vi "Update Value Control.vi"(0 "Session In":T2, 1 "Force update?":bool, 5 "Tree Control In":refnum<vi>, 7 "Tab Control Ref In":T1, 11 "error in (no error)":errorcluster) -> (4 "Session Out":T2, 6 "Tree Control Out":refnum<vi>, 8 "Units":string, 10 "Tooltip":string, 15 "error out":errorcluster)   [LabVIEW 2009, in "IMAQdx Cam.lvclass"]
doc: "The Update Value Control subVI determines the type of the attribute selected, displays the corresponding tab in the tab control, sets the current value of the control, sets the minimum and maximum of the control (for numerics), and disables the control if the attribute is not writables."
uses:
  IMAQdx Cam.lvclass
  <vilib>/userDefined/High Color/IMAQdx.ctl
  <vilib>/vision/driver/IMAQdx.llb/IMAQdx Attribute Type.ctl
  <vilib>/vision/driver/NI_Vision_Acquisition_Software.lvlib
  C:/Program Files/National Instruments/LabVIEW 2009/resource/objmgr/imaqdx.rc
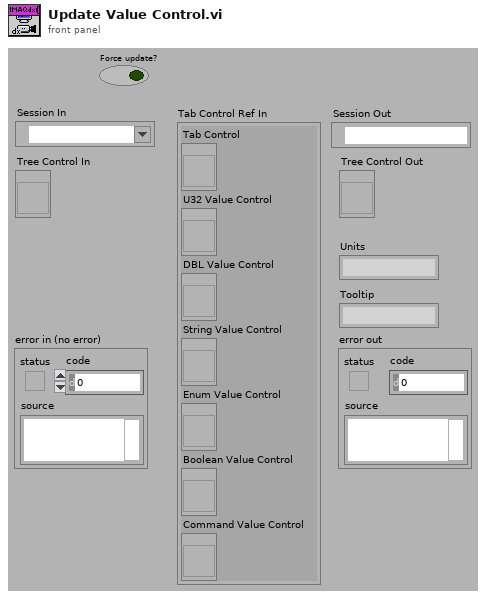
[diagram p1: front panel]
types:
  T1 = cluster{"Tab Control":refnum<vi>, "U32 Value Control":refnum<vi>, "DBL Value Control":refnum<vi>, "String Value Control":refnum<vi>, "Enum Value Control":refnum<vi>, "Boolean Value Control":refnum<vi>, "Command Value Control":refnum<vi>}
  T2 = typedef "IMAQdx.ctl" = refnum<k21>
  T3 = typedef "NI_Vision_Acquisition_Software.lvlib/IMAQdx Attribute Type.ctl" = enum32{"U32", "I64", "DBL", "String", "Enum", "Bool", "Command"}
  T4 = enum32{"U32", "DBL", "String", "Enum", "Bool", "Command"}
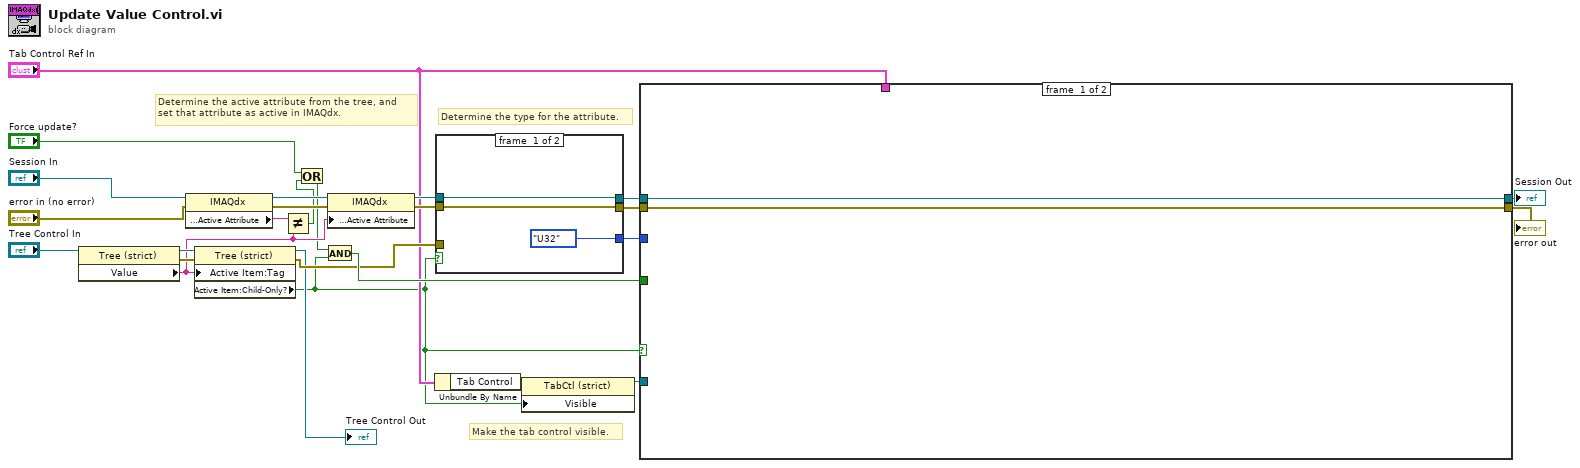
[diagram p0: block diagram]
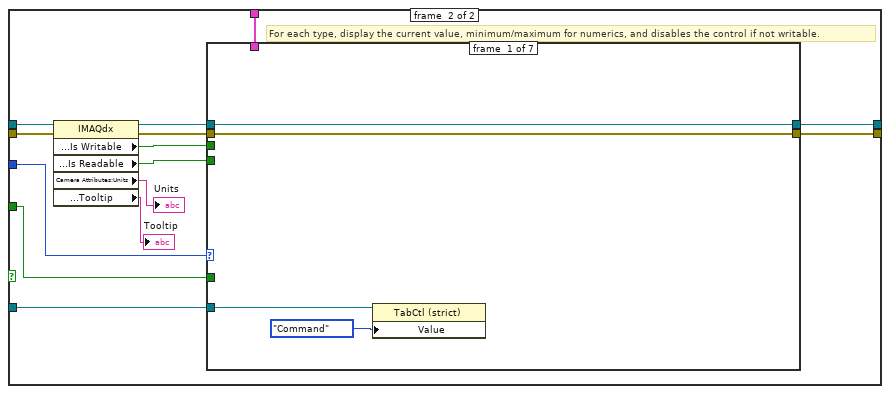
[diagram p2: hidden frame]
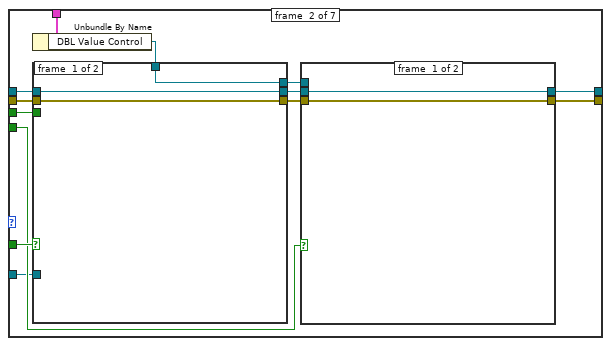
[diagram p3: hidden frame]
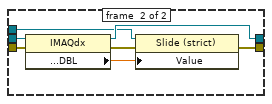
[diagram p4: hidden frame]
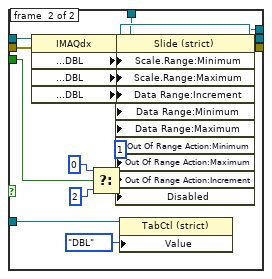
[diagram p5: hidden frame]
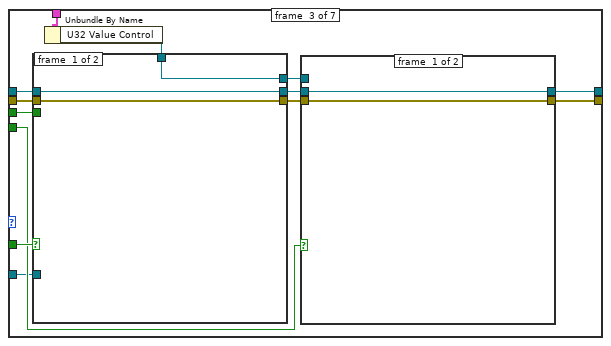
[diagram p6: hidden frame]
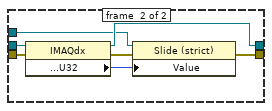
[diagram p7: hidden frame]
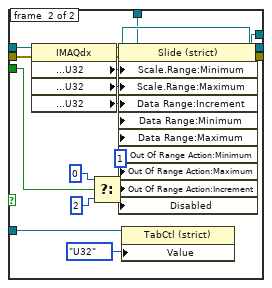
[diagram p8: hidden frame]
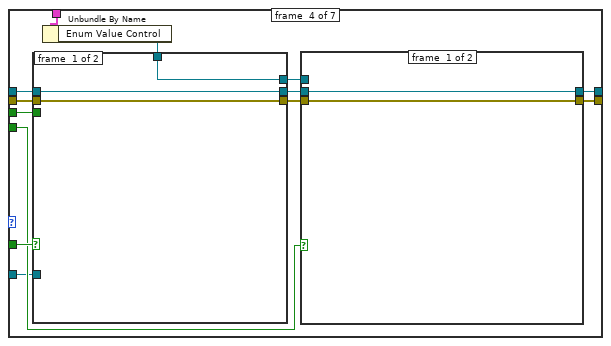
[diagram p9: hidden frame]
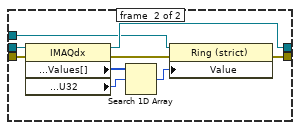
[diagram p10: hidden frame]
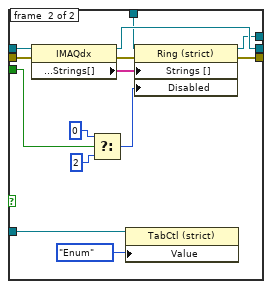
[diagram p11: hidden frame]
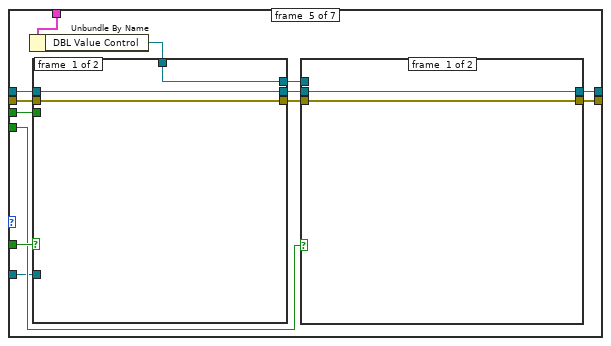
[diagram p12: hidden frame]
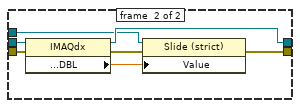
[diagram p13: hidden frame]
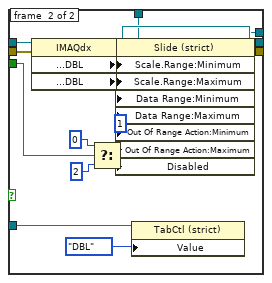
[diagram p14: hidden frame]
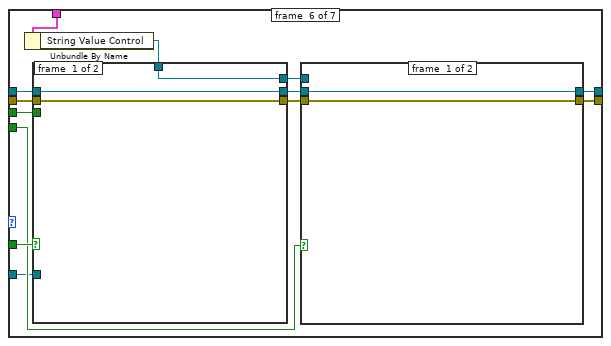
[diagram p15: hidden frame]
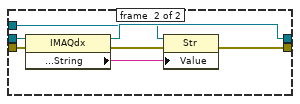
[diagram p16: hidden frame]
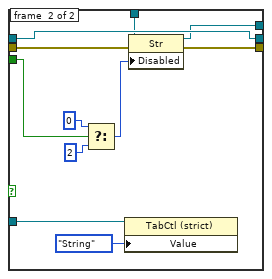
[diagram p17: hidden frame]
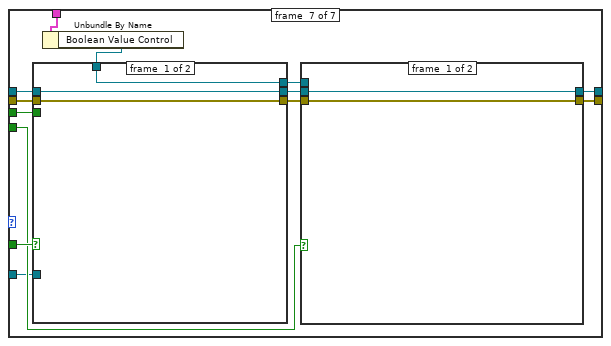
[diagram p18: hidden frame]
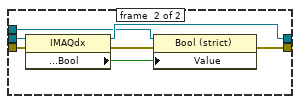
[diagram p19: hidden frame]
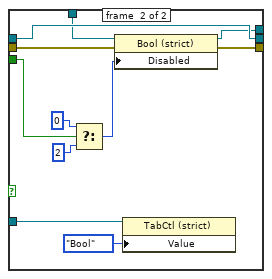
[diagram p20: hidden frame]
diagram:
  # "Make the tab control visible."
  # "Determine the type for the attribute."
  # "Determine the active attribute from the tree, and \nset that attribute as active in IMAQdx."
  n1 = property class="Tree (strict)"(reference="Tree Control In") -> (reference out=w11:refnum<vi>, error out=w10:errorcluster, "Value"=w9:string)  [unwired: 1 in]
  n2 = property class="IMAQdx"(reference="Session In", error in="error in (no error)") -> (reference out=w25:T2, error out=w24:errorcluster, "Camera Attributes:Active Attribute"=w26:string)
  n3 = property class="Tree (strict)"(reference=w11, error in=w10, "Active Item:Tag"=w9) -> (reference out=→"Tree Control Out":refnum<vi>, error out=w17:errorcluster, "Active Item:Child-Only?"=w5:bool)
  n4 = Not Equal?(x=w26, y=w9) -> (x != y?=w3:bool)
  n5 = Or(x="Force update?", y=w3) -> (x .or. y?=w1:bool)
  n6 = And(x=w1, y=w5) -> (x .and. y?=w18:bool)
  n7 = property class="IMAQdx"(reference=w25, error in=w24, "Camera Attributes:Active Attribute"=w9) -> (reference out=w23:T2, error out=w22:errorcluster)
  n8 = Unbundle By Name("Tab Control Ref In") -> ("Tab Control"=w7:refnum<vi>)
  n9 = case shown="True" w5 {
    tunnel: w23 -> [w29 w36]
    tunnel: [w29 w33] -> w20
    tunnel: [IMAQdx_Attribute_Type."U32" ("Attribute Type") w32] -> w19
    tunnel: w22 -> [w27 w31]
    tunnel: [w27 w30] -> w21
    tunnel: w17 -> [_ _]
    frame #0 {
    }
    frame #1 {
      n10 = property class="IMAQdx"(reference=w36, error in=w31) -> (reference out=w33:T2, error out=w30:errorcluster, "Camera Attributes:Type"=w35:u32)
      n11 = Type Cast(type=IMAQdx_Attribute_Type."U32" ("Attribute Type"), x=w35) -> (*(type *) &x=w32:T3)
    }
  }
  n12 = property class="TabCtl (strict)"(reference=w7, "Visible"=w5) -> (reference out=w4:refnum<vi>)  [unwired: 1 in, 1 out]
  n13 = case shown="True" w5 {
    tunnel: w21 -> [w38 w51]
    tunnel: [w38 w43] -> w12
    tunnel: w20 -> [w37 w52]
    tunnel: w19 -> [_ w49]
    tunnel: w18 -> [_ w44]
    tunnel: [w37 w42] -> w13
    tunnel: "Tab Control Ref In" -> [_ w41]
    tunnel: w4 -> [_ w40]
    frame #0 {
    }
    frame #1 {
      # "For each type, display the current value, minimum/maximum for numerics, and disables the control if not writable."
      n14 = property class="IMAQdx"(reference=w52, error in=w51) -> (reference out=w46:T2, error out=w45:errorcluster, "Camera Attributes:Is Writable"=w48:bool, "Camera Attributes:Is Readable"=w47:bool, "Camera Attributes:Units"=→"Units":string, "Camera Attributes:Tooltip"=→"Tooltip":string)
      n15 = case shown="\"DBL\"" w49 {
        tunnel: w48 -> [_ w66 w108 w150 w191 w232 w268]
        tunnel: w47 -> [_ w65 w107 w149 w190 w231 w267]
        tunnel: w46 -> [w55 w69 w111 w153 w194 w235 w271]
        tunnel: w45 -> [w56 w68 w110 w152 w193 w234 w270]
        tunnel: w44 -> [_ w67 w109 w151 w192 w233 w269]
        tunnel: [w56 w62 w104 w146 w187 w228 w264] -> w43
        tunnel: [w55 w61 w103 w145 w186 w227 w263] -> w42
        tunnel: w41 -> [_ w59 w100 w142 w185 w225 w261]
        tunnel: w40 -> [w54 w60 w101 w143 w183 w226 w262]
        frame #0 {
          n16 = property class="TabCtl (strict)"(reference=w54, "Value"=T4."Command" ("Tab Control")) -> ()  [unwired: 1 in, 2 out]
        }
        frame #1 {
          n17 = Unbundle By Name(w59) -> ("DBL Value Control"=w58:refnum<vi>)
          n18 = case shown="True" w67 {
            tunnel: w69 -> [w81 w98]
            tunnel: w68 -> [w80 w97]
            tunnel: [w81 w91] -> w64
            tunnel: [w80 w87] -> w63
            tunnel: w66 -> [_ w96]
            tunnel: w60 -> [_ w93]
            tunnel: w58 -> [w79 w89]
            tunnel: [w79 w88] -> w57
            frame #0 {
            }
            frame #1 {
              w83 = u8 1 ("Out Of Range Action:Maximum")
              n19 = property class="IMAQdx"(reference=w98, error in=w97) -> (reference out=w91:T2, error out=w90:errorcluster, "Camera Attributes:Minimum:DBL"=w85:dbl, "Camera Attributes:Maximum:DBL"=w84:dbl, "Camera Attributes:Increment:DBL"=w82:dbl)
              n20 = Select(t=0, s=w96, f=2) -> (s? t:f=w86:i32)
              n21 = property class="Slide (strict)"(reference=w89, error in=w90, "Scale.Range:Minimum"=w85, "Scale.Range:Maximum"=w84, "Data Range:Increment"=w82, "Data Range:Minimum"=w85, "Data Range:Maximum"=w84, "Out Of Range Action:Minimum"=w83, "Out Of Range Action:Maximum"=w83, "Out Of Range Action:Increment"=w83, "Disabled"=w86) -> (reference out=w88:refnum<vi>, error out=w87:errorcluster)
              n22 = property class="TabCtl (strict)"(reference=w93, "Value"=T4."DBL" ("Tab Control")) -> ()  [unwired: 1 in, 2 out]
            }
          }
          n23 = case shown="True" w65 {
            tunnel: w64 -> [w71 w78]
            tunnel: w63 -> [w70 w77]
            tunnel: [w71 w75] -> w61
            tunnel: [w70 w76] -> w62
            tunnel: w57 -> [_ w73]
            frame #0 {
            }
            frame #1 {
              n24 = property class="IMAQdx"(reference=w78, error in=w77) -> (reference out=w75:T2, error out=w74:errorcluster, "Camera Attributes:Value:DBL"=w72:dbl)
              n25 = property class="Slide (strict)"(reference=w73, error in=w74, "Value"=w72) -> (error out=w76:errorcluster)  [unwired: 1 out]
            }
          }
        }
        frame #2 {
          n26 = Unbundle By Name(w100) -> ("U32 Value Control"=w99:refnum<vi>)
          n27 = case shown="True" w109 {
            tunnel: w111 -> [w123 w140]
            tunnel: w110 -> [w122 w139]
            tunnel: [w123 w134] -> w106
            tunnel: [w122 w132] -> w105
            tunnel: w108 -> [_ w138]
            tunnel: [w121 w131] -> w102
            tunnel: w101 -> [_ w130]
            tunnel: w99 -> [w121 w128]
            frame #0 {
            }
            frame #1 {
              w127 = u8 1 ("Out Of Range Action:Maximum")
              n28 = property class="IMAQdx"(reference=w140, error in=w139) -> (reference out=w134:T2, error out=w135:errorcluster, "Camera Attributes:Minimum:U32"=w125:u32, "Camera Attributes:Maximum:U32"=w124:u32, "Camera Attributes:Increment:U32"=w126:u32)
              n29 = Select(t=0, s=w138, f=2) -> (s? t:f=w133:i32)
              n30 = property class="Slide (strict)"(reference=w128, error in=w135, "Scale.Range:Minimum"=w125, "Scale.Range:Maximum"=w124, "Data Range:Increment"=w126, "Data Range:Minimum"=w125, "Data Range:Maximum"=w124, "Out Of Range Action:Minimum"=w127, "Out Of Range Action:Maximum"=w127, "Out Of Range Action:Increment"=w127, "Disabled"=w133) -> (reference out=w131:refnum<vi>, error out=w132:errorcluster)
              n31 = property class="TabCtl (strict)"(reference=w130, "Value"=T4."U32" ("Tab Control")) -> ()  [unwired: 1 in, 2 out]
            }
          }
          n32 = case shown="True" w107 {
            tunnel: w106 -> [w113 w120]
            tunnel: w105 -> [w112 w119]
            tunnel: [w113 w118] -> w103
            tunnel: [w112 w114] -> w104
            tunnel: w102 -> [_ w115]
            frame #0 {
            }
            frame #1 {
              n33 = property class="IMAQdx"(reference=w120, error in=w119) -> (reference out=w118:T2, error out=w117:errorcluster, "Camera Attributes:Value:U32"=w116:u32)
              n34 = property class="Slide (strict)"(reference=w115, error in=w117, "Value"=w116) -> (error out=w114:errorcluster)  [unwired: 1 out]
            }
          }
        }
        frame #3 {
          n35 = Unbundle By Name(w142) -> ("Enum Value Control"=w141:refnum<vi>)
          n36 = case shown="True" w151 {
            tunnel: w153 -> [w167 w181]
            tunnel: w152 -> [w166 w180]
            tunnel: [w167 w176] -> w148
            tunnel: [w166 w174] -> w147
            tunnel: w150 -> [_ w179]
            tunnel: [w165 w173] -> w144
            tunnel: w143 -> [_ w170]
            tunnel: w141 -> [w165 w168]
            frame #0 {
            }
            frame #1 {
              n37 = property class="IMAQdx"(reference=w181, error in=w180) -> (reference out=w176:T2, error out=w175:errorcluster, "Camera Attributes:Enum:Strings[]"=w171:string[])
              n38 = Select(t=0, s=w179, f=2) -> (s? t:f=w172:i32)
              n39 = property class="TabCtl (strict)"(reference=w170, "Value"=T4."Enum" ("Tab Control")) -> ()  [unwired: 1 in, 2 out]
              n40 = property class="Ring (strict)"(reference=w168, error in=w175, "Strings []"=w171, "Disabled"=w172) -> (reference out=w173:refnum<vi>, error out=w174:errorcluster)
            }
          }
          n41 = case shown="True" w149 {
            tunnel: w148 -> [w155 w164]
            tunnel: w147 -> [w154 w163]
            tunnel: [w155 w158] -> w145
            tunnel: [w154 w160] -> w146
            tunnel: w144 -> [_ w157]
            frame #0 {
            }
            frame #1 {
              n42 = property class="IMAQdx"(reference=w164, error in=w163) -> (reference out=w158:T2, error out=w156:errorcluster, "Camera Attributes:Enum:Values[]"=w162:u32[], "Camera Attributes:Value:U32"=w161:u32)
              n43 = Search 1D Array(1D array=w162, element=w161) -> (index of element=w159:i32)  [unwired: 1 out]
              n44 = property class="Ring (strict)"(reference=w157, error in=w156, "Value"=w159) -> (error out=w160:errorcluster)  [unwired: 1 out]
            }
          }
        }
        frame #4 {
          n45 = Unbundle By Name(w185) -> ("DBL Value Control"=w184:refnum<vi>)
          n46 = case shown="True" w192 {
            tunnel: w194 -> [w206 w222]
            tunnel: w193 -> [w205 w221]
            tunnel: [w206 w217] -> w189
            tunnel: [w205 w212] -> w188
            tunnel: w191 -> [_ w220]
            tunnel: w184 -> [w204 w215]
            tunnel: [w204 w214] -> w182
            tunnel: w183 -> [_ w211]
            frame #0 {
            }
            frame #1 {
              w207 = u8 1 ("Out Of Range Action:Minimum")
              n47 = property class="IMAQdx"(reference=w222, error in=w221) -> (reference out=w217:T2, error out=w216:errorcluster, "Camera Attributes:Minimum:DBL"=w209:dbl, "Camera Attributes:Maximum:DBL"=w208:dbl)
              n48 = Select(t=0, s=w220, f=2) -> (s? t:f=w213:i32)
              n49 = property class="Slide (strict)"(reference=w215, error in=w216, "Scale.Range:Minimum"=w209, "Scale.Range:Maximum"=w208, "Data Range:Minimum"=w209, "Data Range:Maximum"=w208, "Out Of Range Action:Minimum"=w207, "Out Of Range Action:Maximum"=w207, "Disabled"=w213) -> (reference out=w214:refnum<vi>, error out=w212:errorcluster)
              n50 = property class="TabCtl (strict)"(reference=w211, "Value"=T4."DBL" ("Tab Control")) -> ()  [unwired: 1 in, 2 out]
            }
          }
          n51 = case shown="True" w190 {
            tunnel: w189 -> [w196 w203]
            tunnel: w188 -> [w195 w202]
            tunnel: [w196 w201] -> w186
            tunnel: [w195 w199] -> w187
            tunnel: w182 -> [_ w198]
            frame #0 {
            }
            frame #1 {
              n52 = property class="IMAQdx"(reference=w203, error in=w202) -> (reference out=w201:T2, error out=w200:errorcluster, "Camera Attributes:Value:DBL"=w197:dbl)
              n53 = property class="Slide (strict)"(reference=w198, error in=w200, "Value"=w197) -> (error out=w199:errorcluster)  [unwired: 1 out]
            }
          }
        }
        frame #5 {
          n54 = Unbundle By Name(w225) -> ("String Value Control"=w224:refnum<vi>)
          n55 = case shown="True" w233 {
            tunnel: w235 -> [w247 w253]
            tunnel: w234 -> [w246 w251]
            tunnel: [w247 w253] -> w230
            tunnel: [w246 w250] -> w229
            tunnel: w232 -> [_ w258]
            tunnel: w226 -> [_ w255]
            tunnel: w224 -> [w245 w252]
            tunnel: [w245 w248] -> w223
            frame #0 {
            }
            frame #1 {
              n56 = Select(t=0, s=w258, f=2) -> (s? t:f=w249:i32)
              n57 = property class="TabCtl (strict)"(reference=w255, "Value"=T4."String" ("Tab Control")) -> ()  [unwired: 1 in, 2 out]
              n58 = property class="Str"(reference=w252, error in=w251, "Disabled"=w249) -> (reference out=w248:refnum<vi>, error out=w250:errorcluster)
            }
          }
          n59 = case shown="True" w231 {
            tunnel: w230 -> [w237 w244]
            tunnel: w229 -> [w236 w243]
            tunnel: [w237 w242] -> w227
            tunnel: [w236 w240] -> w228
            tunnel: w223 -> [_ w238]
            frame #0 {
            }
            frame #1 {
              n60 = property class="IMAQdx"(reference=w244, error in=w243) -> (reference out=w242:T2, error out=w241:errorcluster, "Camera Attributes:Value:String"=w239:string)
              n61 = property class="Str"(reference=w238, error in=w241, "Value"=w239) -> (error out=w240:errorcluster)  [unwired: 1 out]
            }
          }
        }
        frame #6 {
          n62 = Unbundle By Name(w261) -> ("Boolean Value Control"=w260:refnum<vi>)
          n63 = case shown="True" w269 {
            tunnel: w271 -> [w283 w289]
            tunnel: w270 -> [w282 w286]
            tunnel: [w283 w289] -> w266
            tunnel: [w282 w285] -> w265
            tunnel: w268 -> [_ w294]
            tunnel: w262 -> [_ w291]
            tunnel: w260 -> [w281 w288]
            tunnel: [w281 w287] -> w259
            frame #0 {
            }
            frame #1 {
              n64 = Select(t=0, s=w294, f=2) -> (s? t:f=w284:i32)
              n65 = property class="Bool (strict)"(reference=w288, error in=w286, "Disabled"=w284) -> (reference out=w287:refnum<vi>, error out=w285:errorcluster)
              n66 = property class="TabCtl (strict)"(reference=w291, "Value"=T4."Bool" ("Tab Control")) -> ()  [unwired: 1 in, 2 out]
            }
          }
          n67 = case shown="True" w267 {
            tunnel: w266 -> [w273 w280]
            tunnel: w265 -> [w272 w279]
            tunnel: [w273 w278] -> w263
            tunnel: [w272 w276] -> w264
            tunnel: w259 -> [_ w274]
            frame #0 {
            }
            frame #1 {
              n68 = property class="IMAQdx"(reference=w280, error in=w279) -> (reference out=w278:T2, error out=w277:errorcluster, "Camera Attributes:Value:Bool"=w275:bool)
              n69 = property class="Bool (strict)"(reference=w274, error in=w277, "Value"=w275) -> (error out=w276:errorcluster)  [unwired: 1 out]
            }
          }
        }
      }
    }
  }
  "Session Out" <- w13
  "error out" <- w12
